vi "EnQ Msg Q DVR.vi"(6 "Priority Msg?":bool, 9 "Msg":refnum<class "Msg.lvclass">, 10 "Msg Q DVR":refnum<data-value>) -> (0 "error out":errorcluster)   [LabVIEW 2021, in "LVCAM.lvlib" / "Self Actor.lvclass"]
uses:
  Self Actor.lvclass
  Msg/Msg.lvclass
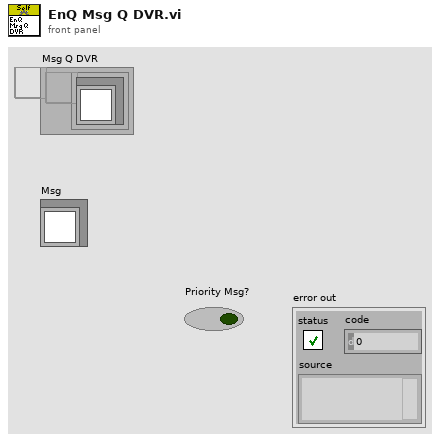
[diagram p1: front panel]
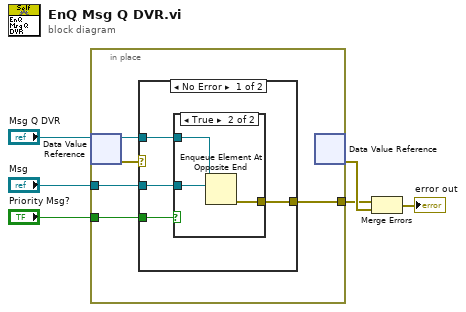
[diagram p0: block diagram]
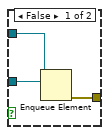
[diagram p2: hidden frame]
diagram:
  n1 = in-place {
    in-place-border: "Msg" -> [w11]
    in-place-border: "Priority Msg?" -> [w10]
    in-place-border: [w9] -> w1
    n2 = in-place-dvr #1("Msg Q DVR") -> (w8:refnum<queue>, w7:errorcluster)
    n3 = case shown="No Error" w7 {
      selector: w7 -> [_ w22]
      tunnel: w11 -> [w15 _]
      tunnel: w10 -> [w14 _]
      tunnel: [w13 w22] -> w9
      tunnel: w8 -> [w12 _]
      frame No Error {
        n4 = case shown="True" w14 {
          tunnel: [w18 w19] -> w13
          tunnel: w12 -> [w17 w21]
          tunnel: w15 -> [w16 w20]
          frame False {
            n5 = Enqueue Element(queue=w17, element=w16) -> (error out=w18:errorcluster)  [unwired: 2 in, 2 out]
          }
          frame True {
            n6 = Enqueue Element At Opposite End(queue=w21, element=w20) -> (error out=w19:errorcluster)  [unwired: 2 in, 2 out]
          }
        }
      }
      frame Error {
      }
    }
    n7 = in-place-dvr #1() -> (w2:errorcluster)  [unwired: 1 in, 1 out]
  }
  n8 = Merge Errors(w1, w2) -> (→"error out":errorcluster)
